vi "GetBuffer.vi"(8 "error in (no error)":errorcluster, 11 "name":string) -> (0 "error out":errorcluster, 3 "DVRBuffer":T1)   [LabVIEW 2017, in "DVRBuffer.lvlib"]
uses:
  <vilib>/addons/InsightCM/Devices/Shared/Common/DVRBuffer/DVRBuffer.lvlib
  <vilib>/addons/InsightCM/Devices/Shared/Common/DVRBuffer/controls/DVRBuffer.ctl
  <vilib>/addons/InsightCM/Devices/Shared/Common/DVRBuffer/controls/DVRElement.ctl
  <vilib>/addons/PointValueMap/subVIs/Point_Read_variant.vi
  <vilib>/addons/PointValueMap/PointValueMap.lvlib
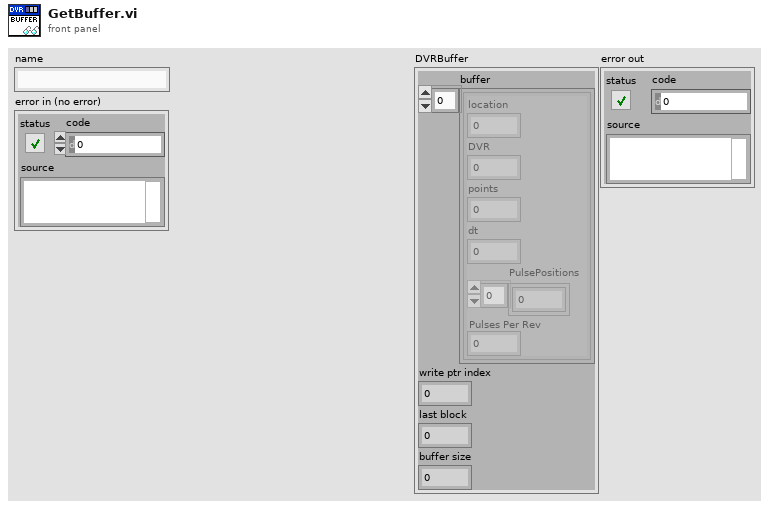
[diagram p1: front panel]
types:
  T1 = typedef "DVRBuffer.lvlib/DVRBuffer.ctl" = cluster{"buffer":T2[], "write ptr index":i32, "last block":u32, "buffer size":u32}
  T2 = typedef "DVRBuffer.lvlib/DVRElement.ctl" = cluster{"location":u32, "DVR":u32, "points":i32, "dt":dbl, "PulsePositions":dbl[], "Pulses Per Rev":dbl}
  T3 = typedef "PointValueMap.lvlib/PointMap.ctl" = refnum<data-value>
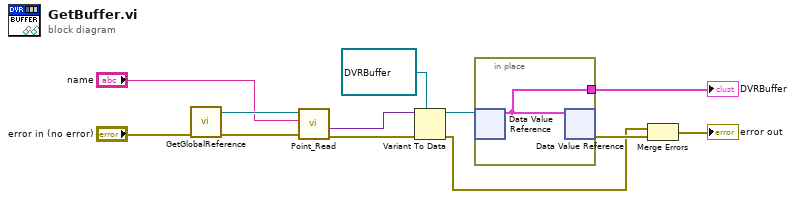
[diagram p0: block diagram]
diagram:
  n1 = call <vilib>:"GetGlobalReference.vi"("error in (no error)"="error in (no error)") -> ("error out"=w11:errorcluster, "reference"=w12:T3)  [unwired: 9 in]
  n2 = call-poly <vilib>:"Point_Read.vi"("Error In"=w11, "Tag"="name", "Map"=w12) -> ("Error Out"=w8:errorcluster, "Value"=w9:variant)  [unwired: 3 in, 4 out]
  n3 = Variant To Data(error in=w8, type=refnum<data-value> refnum ("data value reference"), Variant=w9) -> (data=w6:refnum<data-value>, error out=w3:errorcluster)
  n4 = in-place {
    in-place-border: [w13] -> w5
    n5 = in-place-dvr #1(w6) -> (w13:T1)  [unwired: 1 out]
    n6 = in-place-dvr #1(w13) -> (w4:errorcluster)  [unwired: 1 out]
  }
  "DVRBuffer" <- w5
  n7 = Merge Errors(w3, w4) -> (→"error out":errorcluster)
